vi "Unescape Python String.vi"(10 "Escaped Python String":string) -> (2 "Unescaped String":string)   [LabVIEW 2020, in "jki_python_data_tools.lvlib"]
uses:
  jki_python_data_tools.lvlib
  9d250df1-c27a-4e71-b21f-beb3fd7fe870.vi
  9d250df1-c27a-4e71-b21f-beb3fd7fe870.vi/b0178052-0c48-4c9a-874f-40b592e34ac5.vi
panel:
  # "Copyright © 2003-2009 JKI. All rights reserved.\n\nAuthor: Jim Kring [jim.kring@jameskring.com]\n\nThis library is provided \"AS IS\" ,WITHOUT WARRANTIES OR \nCONDITIONS OF ANY KIND, either express or implied.\n\nJames Kring, Inc. -- http://www.jameskring.com"
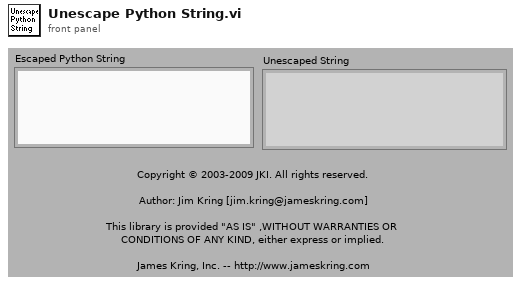
[diagram p1: front panel]
types:
  T1 = cluster{"Char ('\\' Codes Display)":string, "Escape Code (Normal Display)":string}[]
  T2 = cluster{"Escape Code (Normal Display)":string, "Char ('\\' Codes Display)":string}
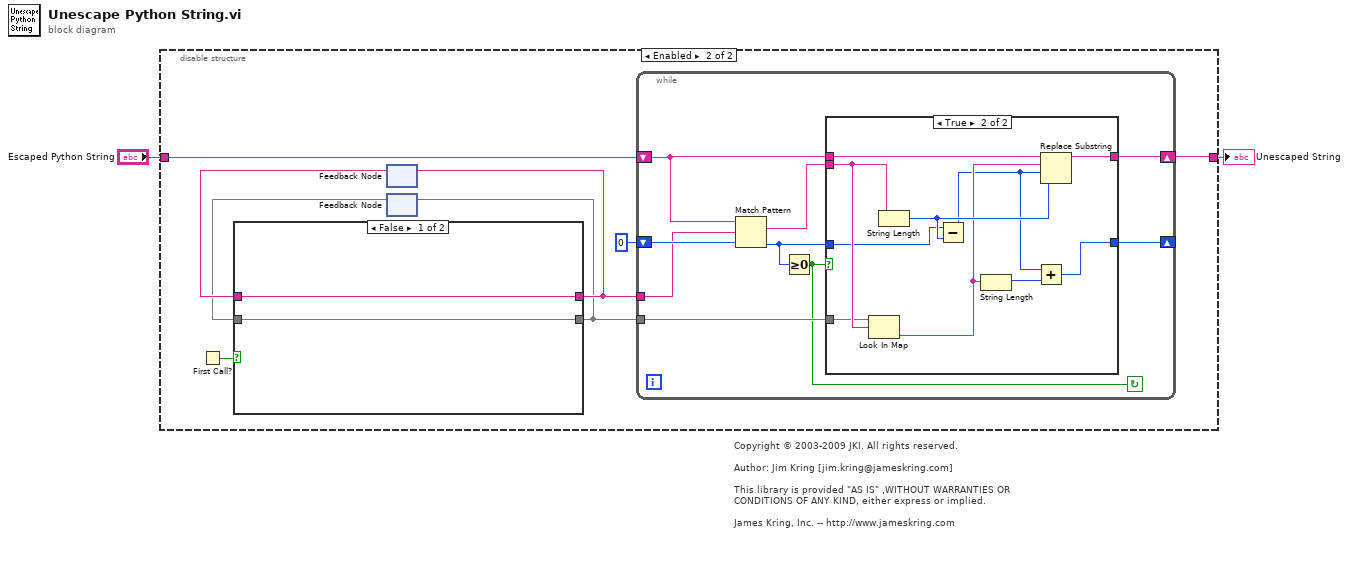
[diagram p0: block diagram]
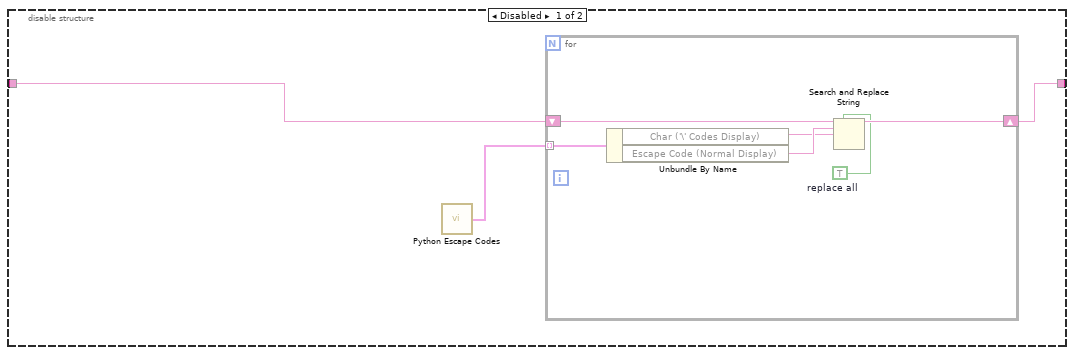
[diagram p2: hidden frame]
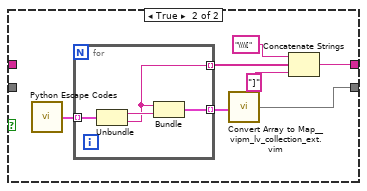
[diagram p3: hidden frame]
diagram:
  # "Copyright © 2003-2009 JKI. All rights reserved.\n\nAuthor: Jim Kring [jim.kring@jameskring.com]\n\nThis library is provided \"AS IS\" ,WITHOUT WARRANTIES OR \nCONDITIONS OF ANY KIND, either express or implied.\n\nJames Kring, Inc. -- http://www.jameskring.com"
  n1 = disable-structure shown="Enabled" {
    disable-tunnel: [w5 w18] -> w2
    disable-tunnel: "Escaped Python String" -> [w4 w19]
    frame Disabled {
      n2 = call "Python Escape Codes.vi"() -> ("Python Escape Codes"=w3:T1)
      n3 = for {
        shift-right: [w10] -> w5
        shift-left: w4 -> [w11]
        tunnel: w3 -> [w8] mode=indexing
        w9 = TRUE  # replace all
        n4 = Unbundle By Name(w8) -> ("Char ('\\' Codes Display)"=w6:string, "Escape Code (Normal Display)"=w7:string)
        n5 = Search and Replace String(replace all?=w9, input string=w11, search string=w7, replace string=w6) -> (result string=w10:string)  [unwired: 4 in, 3 out]
      }
    }
    frame Enabled {
      n6 = First Call?() -> (First Call?: T/F=w16:bool)
      n7 = feedback #1() -> (w13:string)  [unwired: 1 in]
      n8 = feedback #2() -> (w12:map{string, string})  [unwired: 1 in]
      n9 = case shown="False" w16 {
        tunnel: [w21 w23] -> w15
        tunnel: [w20 w22] -> w14
        tunnel: w13 -> [w21 _]
        tunnel: w12 -> [w20 _]
        frame False {
        }
        frame True {
          n10 = call "Python Escape Codes.vi"() -> ("Python Escape Codes"=w26:T1)
          n11 = for {
            tunnel: w26 -> [w32] mode=indexing
            tunnel: [w30] -> w27 mode=indexing
            tunnel: [w29] -> w28 mode=indexing
            n12 = Unbundle(w32) -> ("Char ('\\' Codes Display)"=w31:string, "Escape Code (Normal Display)"=w29:string)
            n13 = Bundle("Escape Code (Normal Display)"=w29, "Char ('\\' Codes Display)"=w31) -> (w30:T2)  [unwired: 1 in]
          }
          n14 = call "Convert Array to Map__vipm_lv_collection_ext.vim"("array"=w27) -> ("map"=w22:map{string, string})  [unwired: 6 in]
          n15 = Concatenate Strings("\\\\[" ("regular expression"), w28, "]" ("regular expression")) -> (w23:string)
        }
      }
      n16 = feedback-in #1(w15) -> ()
      n17 = feedback-in #2(w14) -> ()
      n18 = while {
        shift-right: [w37] -> _
        shift-left: 0 ("offset past match") -> [w41]
        tunnel: w14 -> [w38]
        tunnel: w15 -> [w36]
        shift-right: [w40] -> w18
        shift-left: w19 -> [w33]
        stop <- w34 continue-if-true
        n19 = Match Pattern(string=w33, regular expression=w36, offset (0)=w41) -> (match substring=w39:string, offset past match=w35:i32)  [unwired: 2 out]
        n20 = Greater Or Equal To 0?(x=w35) -> (x >= 0?=w34:bool)
        n21 = case shown="True" w34 {
          tunnel: w33 -> [w43 w53]
          tunnel: [w43 w52] -> w40
          tunnel: w39 -> [_ w50]
          tunnel: w38 -> [_ w49]
          tunnel: [w42 w45] -> w37
          tunnel: w35 -> [w42 w44]
          frame False {
          }
          frame True {
            n22 = Look In Map(map=w49, key=w50) -> (value=w48:string)  [unwired: 1 in, 1 out]
            n23 = String Length(string=w50) -> (length=w51:i32)
            n24 = Subtract(x=w44, y=w51) -> (x-y=w47:i32)
            n25 = String Length(string=w48) -> (length=w46:i32)
            n26 = Add(x=w47, y=w46) -> (x+y=w45:i32)
            n27 = Replace Substring(2:w51, 3:w47, 4:w48, 5:w53) -> (1:w52:string)  [unwired: 1 out]
          }
        }
      }
    }
  }
  "Unescaped String" <- w2
